vi "Move SC Motor 2(SubVI).vi"(0 "String":string, 1 "error out":errorcluster, 2 "Speed":i32, 3 "VISA resource name out":refnum<visa-resource-name>, 4 "Position":i32, 5 "Output":refnum<vi>, 6 "Input":refnum<vi>) -> ()   [LabVIEW 2013]
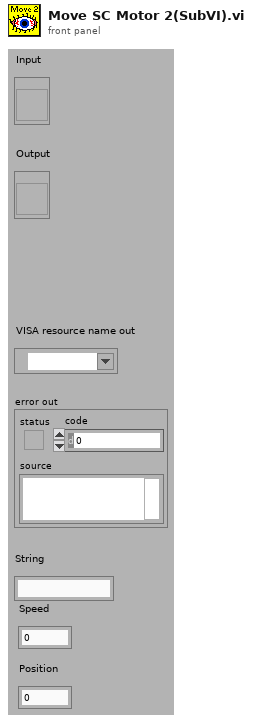
[diagram p1: front panel]
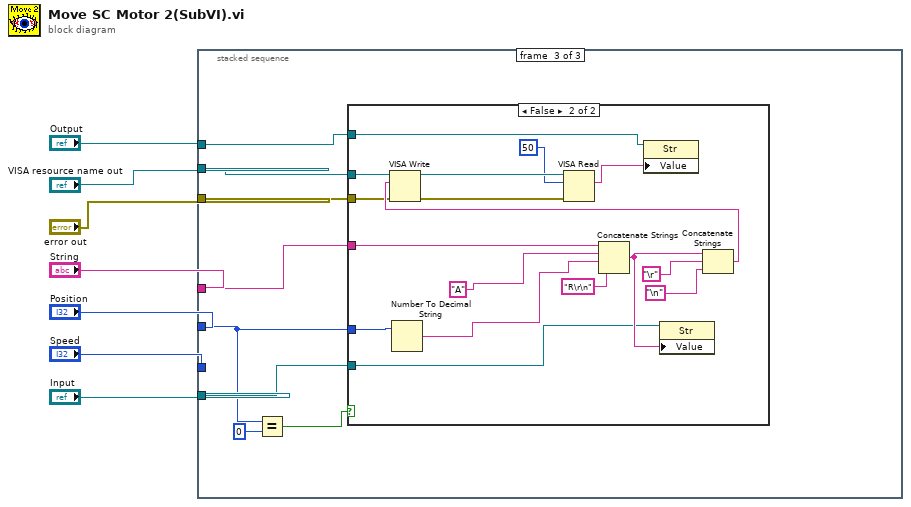
[diagram p0: block diagram]
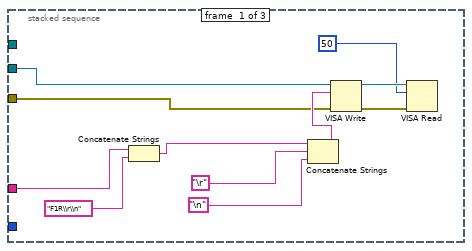
[diagram p2: hidden frame]
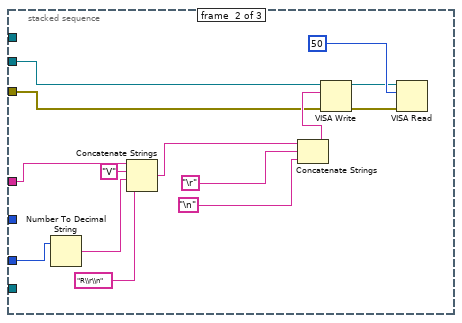
[diagram p3: hidden frame]
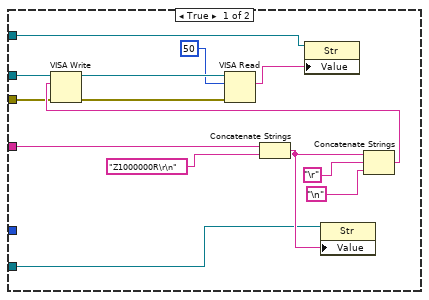
[diagram p4: hidden frame]
diagram:
  n1 = stacked-sequence {
    tunnel: "VISA resource name out" -> [w12 w25 w40]
    tunnel: "error out" -> [w11 w26 w39]
    tunnel: "String" -> [w10 w21 w38]
    tunnel: "Input" -> [_ _ w37]
    tunnel: "Output" -> [_ _ w36]
    tunnel: "Speed" -> [_ w22 _]
    tunnel: "Position" -> [_ _ w33]
    frame #0 {
      n2 = Concatenate Strings(w10, "F1R\\r\\n") -> (w8:string)
      n3 = Concatenate Strings(w8, "\r", "\n") -> (w15:string)
      n4 = VISA Write(VISA resource name=w12, write buffer=w15, error in (no error)=w11) -> (VISA resource name out=w17:refnum<visa-resource-name>, error out=w18:errorcluster)  [unwired: 1 out]
      n5 = VISA Read(VISA resource name=w17, byte count=u32 50, error in (no error)=w18) -> ()  [unwired: 4 out]
    }
    frame #1 {
      n6 = Number To Decimal String(number=w22) -> (decimal integer string=w19:string)  [unwired: 1 in]
      n7 = Concatenate Strings(w21, "V" ("string"), w19, "R\\r\\n") -> (w23:string)
      n8 = Concatenate Strings(w23, "\r", "\n") -> (w30:string)
      n9 = VISA Write(VISA resource name=w25, write buffer=w30, error in (no error)=w26) -> (VISA resource name out=w28:refnum<visa-resource-name>, error out=w27:errorcluster)  [unwired: 1 out]
      n10 = VISA Read(VISA resource name=w28, byte count=u32 50, error in (no error)=w27) -> ()  [unwired: 4 out]
    }
    frame #2 {
      n11 = Equal?(x=w33, y=0) -> (x = y?=w35:bool)
      n12 = case shown="False" w35 {
        tunnel: w40 -> [w49 w65]
        tunnel: w39 -> [w48 w64]
        tunnel: w38 -> [w47 w61]
        tunnel: w37 -> [w43 w57]
        tunnel: w36 -> [w42 w56]
        tunnel: w33 -> [_ w55]
        frame True {
          n13 = Concatenate Strings(w47, "Z1000000R\r\n" ("string")) -> (w45:string)
          n14 = property class="Str"(reference=w43, "Value"=w45) -> ()  [unwired: 1 in, 2 out]
          n15 = Concatenate Strings(w45, "\r", "\n") -> (w51:string)
          n16 = VISA Write(VISA resource name=w49, write buffer=w51, error in (no error)=w48) -> (VISA resource name out=w53:refnum<visa-resource-name>, error out=w54:errorcluster)  [unwired: 1 out]
          n17 = VISA Read(VISA resource name=w53, byte count=u32 50, error in (no error)=w54) -> (read buffer=w44:string)  [unwired: 3 out]
          n18 = property class="Str"(reference=w42, "Value"=w44) -> ()  [unwired: 1 in, 2 out]
        }
        frame False {
          n19 = Number To Decimal String(number=w55) -> (decimal integer string=w62:string)  [unwired: 1 in]
          n20 = Concatenate Strings(w61, "A" ("string"), w62, "R\r\n" ("string")) -> (w59:string)
          n21 = property class="Str"(reference=w57, "Value"=w59) -> ()  [unwired: 1 in, 2 out]
          n22 = Concatenate Strings(w59, "\r", "\n") -> (w68:string)
          n23 = VISA Write(VISA resource name=w65, write buffer=w68, error in (no error)=w64) -> (VISA resource name out=w70:refnum<visa-resource-name>, error out=w71:errorcluster)  [unwired: 1 out]
          n24 = VISA Read(VISA resource name=w70, byte count=u32 50, error in (no error)=w71) -> (read buffer=w58:string)  [unwired: 3 out]
          n25 = property class="Str"(reference=w56, "Value"=w58) -> ()  [unwired: 1 in, 2 out]
        }
      }
    }
  }
